vi "Periodic Tasks.vi"(8 "error in (no error)":errorcluster) -> ()   [LabVIEW 2014]
doc: "This VI runs in parallel to other tasks. It can contain as many user-defined periodic loops as you need. These can carry out PID or other sorts of timed response."
uses:
  <vilib>/Rock Robotics/WPI/DriverStation/WPI_DriverStationRobotMode2.ctl
  <vilib>/Utility/file.llb/Write To Spreadsheet File (string).vi
  <vilib>/Utility/file.llb/Write To Spreadsheet File (DBL).vi
  <vilib>/Rock Robotics/WPI/Joystick/WPI_JoystickGetSetRefNum.vi
  Robot Global Data.vi
  <vilib>/Rock Robotics/Network Tables/SD Read Boolean.vi
  <vilib>/Rock Robotics/Network Tables/SD Write Number.vi
  <vilib>/Rock Robotics/Network Tables/NT Write Number.vi
  <vilib>/Rock Robotics/Network Tables/SD Write Numeric Array.vi
  <vilib>/Rock Robotics/Network Tables/NT Read Boolean.vi
  <vilib>/Rock Robotics/Network Tables/NT Write Boolean.vi
  <vilib>/FPGAPlugInAG/roboRIO/niLvFpga_Close_roboRIO.vi
  <vilib>/Rock Robotics/SystemInterfaces/System/FPGA_SystemFPGA Ref Global.vi
  <vilib>/rvi/interface/nirviCloseFPGA/nirviCloseFPGA.xnode
  <vilib>/Rock Robotics/SystemInterfaces/System/FPGA_SystemFRC FPGA Ref.ctl
  <vilib>/Rock Robotics/SystemInterfaces/roboRIO_FPGA_2015_1.0.10.lvbitx
  navX-MXP-LabVIEW/navX-MXP Library/navX-MXP IMU.lvlib
  <vilib>/Rock Robotics/WPI/DriverStation/WPI_DriverStationAllianceInfo.ctl
  <vilib>/Rock Robotics/Network Tables/SD Read Number.vi
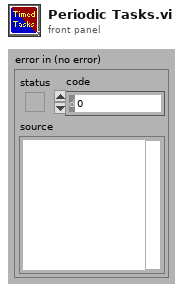
[diagram p1: front panel]
types:
  T1 = typedef "WPI_DriverStationRobotMode2.ctl" = enum16{"Autonomous Disabled", "Autonomous Enabled", "Teleop Disabled", "Teleop Enabled", "Disconnected", "Finish", "Test Disabled", "Test Enabled", "Emergency Stopped"}
  T2 = typedef "WPI_DriverStationPositionInfo.ctl" = enum16{"1", "2", "3"}
  T3 = typedef "WPI_DriverStationAllianceInfo.ctl" = enum16{"Red", "Blue", "Invalid"}
  T4 = typedef "WPI_MotorControlDeviceRef.ctl" = cluster{"DeviceStatus":errorcluster, "Type":T5, "PWM":cluster{"Controller":T6, "PWM Channel":T7, "DeadBand":T8}, "CAN":cluster{"Device Number":u8, "Control Mode":T9, "Semaphore":T10, "Max Vout":dbl, "TalonSRX Control Mode":T11}, "Invert":bool, "TransformRef":T12, "InvTransformRef":T12}
  T5 = typedef "WPI_MotorControlType.ctl" = enum16{"PWM", "CAN", "CANTalonSRX"}
  T6 = typedef "FPGA_TypedefDigitalModule.ctl" = enum16{"Controller 1"}
  T7 = typedef "FPGA_DIOPWMChannel.ctl" = enum8{"PWM 0", "PWM 1", "PWM 2", "PWM 3", "PWM 4", "PWM 5", "PWM 6", "PWM 7", "PWM 8", "PWM 9", "PWM MXP 0", "PWM MXP 1", "PWM MXP 2", "PWM MXP 3", "PWM MXP 4", "PWM MXP 5", "PWM MXP 6", "PWM MXP 7", "PWM MXP 8", "PWM MXP 9", "Invalid"}
  T8 = typedef "WPI_PWMDeadband.ctl" = cluster{"Name":string, "maxPositivePwm":i32, "minPositivePwm":i32, "centerPwm":i32, "maxNegativePwm":i32, "minNegativePwm":i32, "angularRange":u16}
  T9 = typedef "WPI_CANJaguar_ControlMode.ctl" = enum8{"Percent VBus", "Current", "Speed", "Position", "Voltage"}
  T10 = typedef "Semaphore RefNum" = refnum<k1>
  T11 = typedef "WPI_CANTalonSRX_APIControlMode.ctl" = enum8{"Percent VBus", "Speed", "Position", "Slave", "Unchanged / Invalid"}
  T12 = typedef "WPI_PWMTransform_ConPane.ctl" = refnum<vi>
  T13 = cluster{"FL Steering":T4, "FR Steering":T4, "RL Steering":T4, "RR Steering":T4}
  T14 = cluster{"FL Speed":T4, "FR Speed":T4, "RL Speed":T4, "RR Speed":T4}
  T15 = typedef "navX-MXP IMU.lvlib/navX Device TypeDef.ctl" = cluster{"navX Interface Protocol":T16, "navX Interface Protocol TypeDefs":cluster{"SPIDevRef":T17, "I2CDevRef":T19}, "navX System Information":cluster{"Board Information":T21, "Status":T22, "Offsets":T26}, "navX Common Information":cluster{"Update Rate (4Hz-60Hz)":T27, "refnum name":string, "error":errorcluster}}
  T16 = typedef "navX-MXP IMU.lvlib/navX Interface Protocol.ctl" = enum16{"SPI", "I2C"}
  T17 = typedef "WPI_SPIDevRef.ctl" = cluster{"DevStatus":errorcluster, "Handle":i32, "Controller":T6, "SPI Bus":T18}
  T18 = typedef "spi_bus.ctl" = enum16{"SPI On-Board, CS0", "SPI On-Board, CS1", "SPI On-Board, CS2", "SPI On-Board, CS3", "SPI MXP", "Invalid"}
  T19 = typedef "WPI_I2CDevRef.ctl" = cluster{"DevStatus":errorcluster, "Controller":T6, "Device Address":u8, "Handle":i32, "I2C Bus":T20}
  T20 = typedef "i2c_bus.ctl" = enum16{"I2C On-Board", "I2C MXP", "Invalid"}
  T21 = typedef "navX-MXP IMU.lvlib/navX Board Information.ctl" = cluster{"WhoAmI (50 | 0x32)":u8, "Board Revision":u8, "Firmware Major Version":u8, "Firmware Minor Version":u8}
  T22 = typedef "navX-MXP IMU.lvlib/navX Status Data.ctl" = cluster{"Update Rate Hz":u8, "Accelerometer Full-Scale Range":u8, "Gyro Full-Scale Range":u16, "NAVX_OP_STATUS":T23, "NAVX_CAL_STATUS":T24, "NAVX_SELFTEST_STATUS":u8, "NAVX_SENSOR_STATUS":T25}
  T23 = typedef "navX-MXP IMU.lvlib/navX NAVX_OP_STATUS.ctl" = u8
  T24 = typedef "navX-MXP IMU.lvlib/navX NAVX_CAL_STATUS.ctl" = u8
  T25 = typedef "navX-MXP IMU.lvlib/navX NAVX_SENSOR_STATUS.ctl" = cluster{"MOVING":bool, "YAW_STABLE":bool, "MAG_DISTURBANCE":bool, "ALTITUDE_VALID":bool, "SEALEVEL_PRESS_SET":bool, "FUSED_HEADING_VALID":bool}
  T26 = typedef "navX-MXP IMU.lvlib/navX Offsets Data.ctl" = cluster{"Yaw":dbl, "Quat W":dbl, "Quat X":dbl, "Quat Y":dbl, "Quat Z":dbl}
  T27 = typedef "navX-MXP IMU.lvlib/navX Update Rate.ctl" = u8
  T28 = typedef "navX-MXP IMU.lvlib/navX YPRH Data.ctl" = cluster{"Yaw":dbl, "Pitch":dbl, "Roll":dbl, "Heading":dbl}
  T29 = typedef "WPI_CANTalonSRX_GlobalStatus.ctl" = cluster{"Applied Throttle":dbl, "Module Enabled":bool, "CAN Error":errorcluster, "Closed Loop Error":dbl, "Forward Limit Switch Closed":bool, "Reverse Limit Switch Closed":bool, "Sensor Position":dbl, "Sensor Velocity":dbl, "Current":dbl, "Sticky Fault - Over Temp":bool, "Sticky Fault - Under Voltage":bool, "Sticky Fault - Forward Limit":bool, "Sticky Fault - Reverse Limit":bool, "Sticky Fault - Forward Soft Limit":bool, "Sticky Fault - Reverse Soft Limit":bool, "Brake is Enabled":bool, "Encoder Position":dbl, "Encoder Velocity":dbl, "Encoder Index Count":dbl, "Encoder A Pin State":bool, "Encoder B Pin State":bool, "Encoder Index Pin State":bool, "Analog In":dbl, "Analog In Velocity":dbl, "Temperature (C)":dbl, "Battery Voltage":dbl}
  T30 = cluster{"[0]":dbl, "[1]":dbl, "[2]":dbl, "[3]":dbl}
  T31 = typedef "FPGA_SystemFRC FPGA Ref.ctl" = refnum<k20>
  T32 = cluster{"refnum name":string, "refnum name":string, "refnum name":string, "refnum name":string}
  T33 = typedef "WPI_AnalogChannelDevRef.ctl" = cluster{"DevStatus":errorcluster, "Controller":T34, "Analog Channel":T35}
  T34 = typedef "FPGA_TypedefAnalogModule.ctl" = enum16{"Controller 1"}
  T35 = typedef "FPGA_AIChannel.ctl" = enum8{"AI 0", "AI 1", "AI 2", "AI 3", "AI MXP 0", "AI MXP 1", "AI MXP 2", "AI MXP 3", "Invalid"}
  T36 = typedef "WPI_JoystickDevRef.ctl" = cluster{"Device":T37}
  T37 = typedef "WPI_JoystickDeviceEnum.ctl" = enum16{"USB 0", "USB 1", "USB 2", "USB 3", "USB 4", "USB 5"}
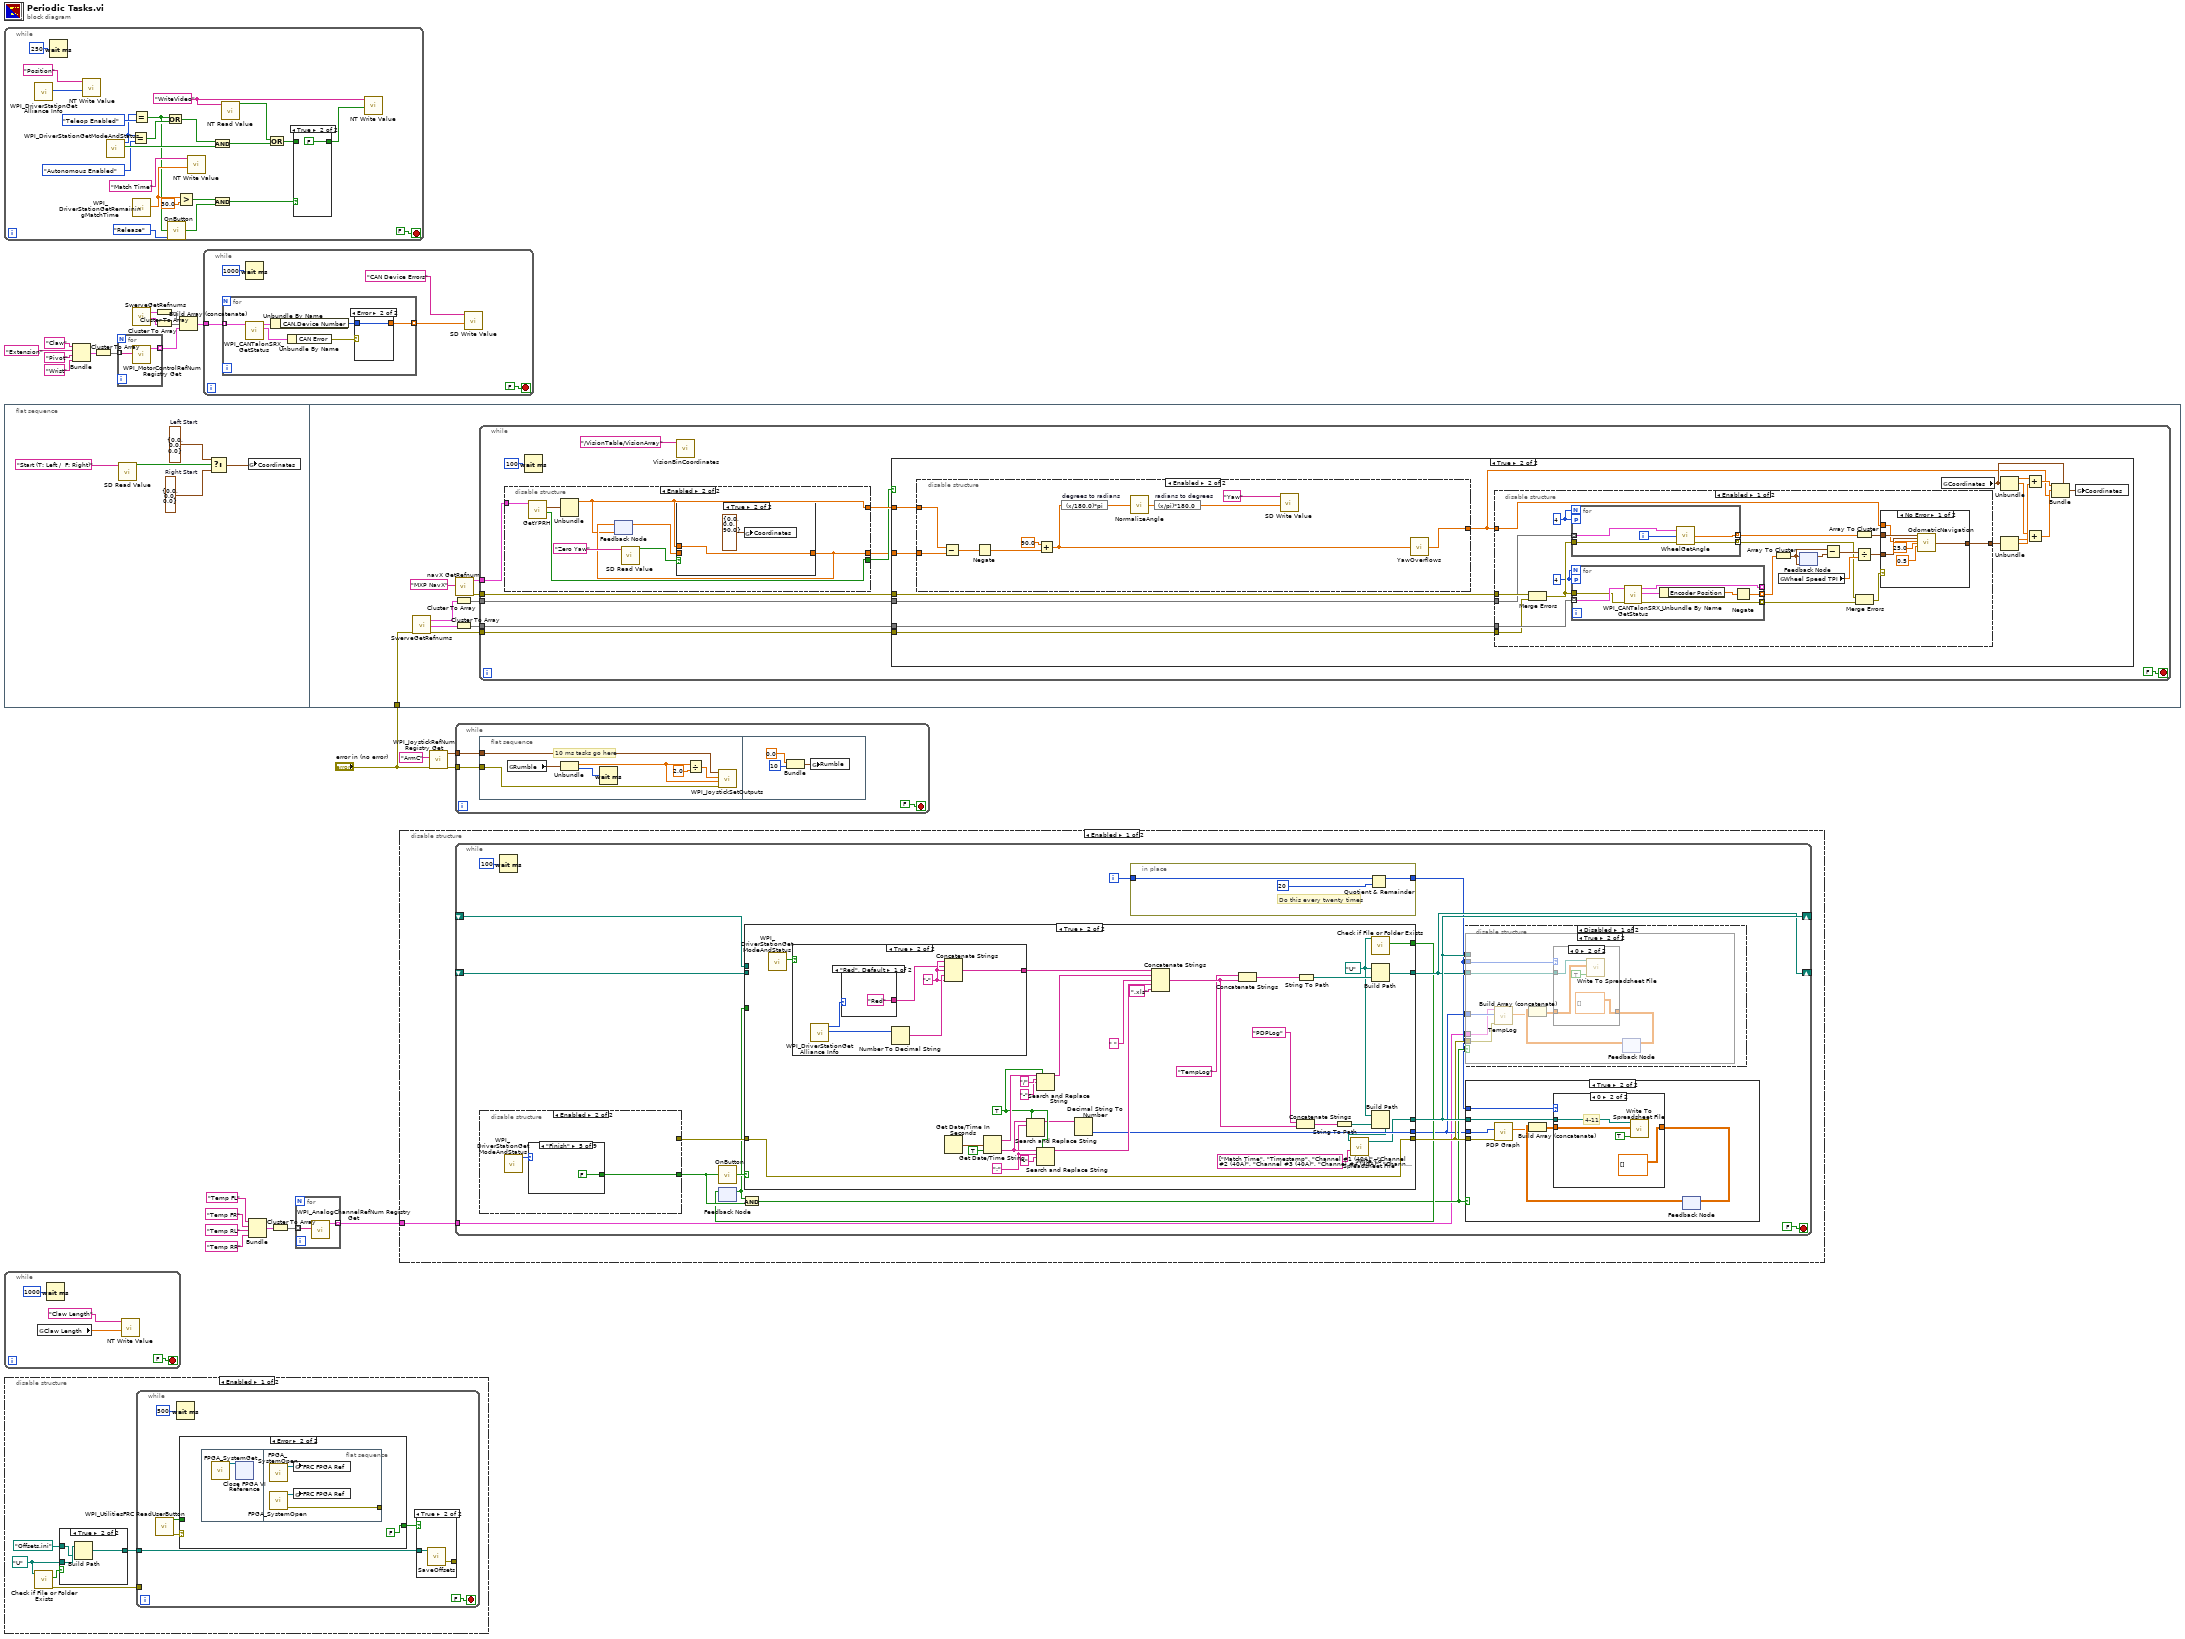
[diagram p0: block diagram]
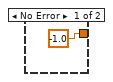
[diagram p3: hidden frame]
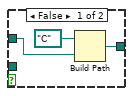
[diagram p4: hidden frame]
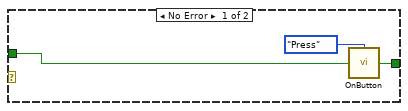
[diagram p5: hidden frame]
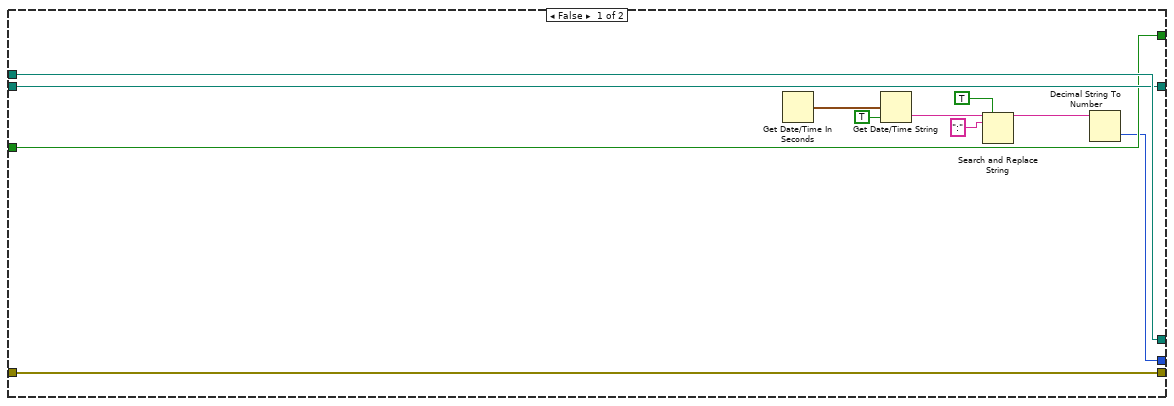
[diagram p11: hidden frame]
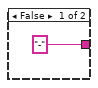
[diagram p12: hidden frame]
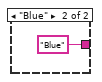
[diagram p13: hidden frame]
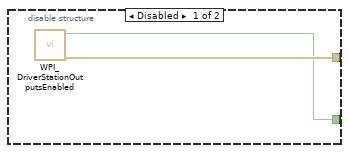
[diagram p16: hidden frame]
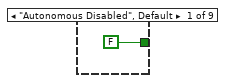
[diagram p17: hidden frame]
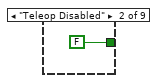
[diagram p18: hidden frame]
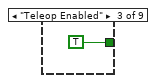
[diagram p19: hidden frame]
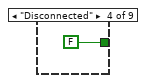
[diagram p20: hidden frame]
diagram:
  n1 = while {
    stop <- FALSE stop-if-true
    w43 = "WriteVideo" ("Name")
    n2 = call <vilib>:"WPI_DriverStationGet Alliance Info.vi"() -> ("Position"=w42:T2)  [unwired: 10 in, 1 out]
    n3 = Wait (ms)(milliseconds to wait=250) -> ()  [unwired: 1 out]
    n4 = call-poly <vilib>:"NT Write Value.vi"("Numeric"=w42, "Name"="Position") -> ()  [unwired: 9 in, 1 out]
    n5 = call <vilib>:"WPI_DriverStationGetModeAndStatus.vi"() -> ("FMS Attached"=w44:bool, "Robot Mode"=w28:T1)  [unwired: 10 in]
    n6 = Equal?(x=w28, y=WPI_DriverStationRobotMode2."Autonomous Enabled") -> (x = y?=w25:bool)
    n7 = Equal?(x=w28, y=WPI_DriverStationRobotMode2."Teleop Enabled" ("Robot Mode")) -> (x = y?=w24:bool)
    n8 = call <vilib>:"WPI_DriverStationGetRemainingMatchTime.vi"() -> ("Match Time(s)"=w31:sgl)  [unwired: 10 in, 1 out]
    n9 = Or(x=w24, y=w25) -> (x .or. y?=w26:bool)
    n10 = call "OnButton.vi"("Button"=w24, "Mode"=enum16{"Press", "Release", "Both"}."Release") -> ("Value"=w36:bool)
    n11 = Greater?(x=w31, y=sgl 30.0) -> (0:w33:bool)
    n12 = call-poly <vilib>:"NT Write Value.vi"("Numeric"=w31, "Name"="Match Time") -> ()  [unwired: 9 in, 1 out]
    n13 = And(x=w26, y=w44) -> (x .and. y?=w37:bool)
    n14 = And(x=w33, y=w36) -> (x .and. y?=w34:bool)
    n15 = call-poly <vilib>:"NT Read Value.vi"("Name"=w43) -> ("Boolean"=w38:bool)  [unwired: 9 in, 1 out]
    n16 = Or(x=w38, y=w37) -> (x .or. y?=w39:bool)
    n17 = case shown="True" w34 {
      tunnel: [w47 FALSE] -> w40
      tunnel: w39 -> [w47 _]
      frame False {
      }
      frame True {
      }
    }
    n18 = call-poly <vilib>:"NT Write Value.vi"("Boolean"=w40, "Name"=w43) -> ()  [unwired: 9 in, 1 out]
  }
  n19 = flat-sequence {
    tunnel: "error in (no error)" -> [w62]
    frame #0 {
      w49 = cluster{"X":dbl, "Y":dbl, "Heading":dbl} {"X"=0.0, "Y"=0.0, "Heading"=0.0}  # Left Start
      w50 = cluster{"X":dbl, "Y":dbl, "Heading":dbl} {"X"=0.0, "Y"=0.0, "Heading"=0.0}  # Right Start
      n20 = call-poly <vilib>:"SD Read Value.vi"("Name"="Start (T: Left /  F: Right)") -> ("Boolean"=w52:bool)  [unwired: 8 in, 2 out]
      n21 = Select(t=w49, s=w52, f=w50) -> (s? t:f=w51:cluster{"X":dbl, "Y":dbl, "Heading":dbl})
      n22 = global write "Robot Global Data.vi" "Coordinates"(w51) -> ()
    }
    frame #1 {
      n23 = call "SwerveGetRefnums.vi"("error in (no error)"=w62) -> ("Steering"=w55:T13, "Speed"=w57:T14, "error out"=w56:errorcluster)  [unwired: 8 in, 8 out]
      n24 = Cluster To Array(cluster=w55) -> (array=w54:T4[])
      n25 = Cluster To Array(cluster=w57) -> (array=w58:T4[])
      n26 = call "navX GetRefnum.vi"("refnum name"="MXP NavX") -> ("error out"=w59:errorcluster, "navX Device TypeDef"=w60:T15)  [unwired: 9 in]
      n27 = while {
        tunnel: w60 -> [w70]
        tunnel: w59 -> [w69]
        tunnel: w56 -> [w65]
        tunnel: w58 -> [w66]
        tunnel: w54 -> [w64]
        stop <- FALSE stop-if-true
        n28 = disable-structure shown="Enabled" {
          disable-tunnel: [w76 w77] -> w72
          disable-tunnel: [w75 w82] -> w71
          disable-tunnel: w70 -> [w74 w84]
          disable-tunnel: [_ w79] -> w68
          frame Disabled {
            n29 = call "GetFusedHeading.vi"("navX Device TypeDef"=w74) -> ("Valid?"=w75:bool, "Fused Heading"=w76:dbl)  [unwired: 8 in, 1 out]
          }
          frame Enabled {
            n30 = call "GetYPRH.vi"("navX Device TypeDef"=w84) -> ("Valid?"=w82:bool, "YPRH"=w83:T28)  [unwired: 8 in, 1 out]
            n31 = Unbundle(w83) -> ("Yaw"=w77:dbl)  [unwired: 3 out]
            n32 = feedback #1(w77) -> (w80:dbl)
            n33 = call-poly <vilib>:"SD Read Value.vi"("Name"="Zero Yaw") -> ("Boolean"=w78:bool)  [unwired: 8 in, 2 out]
            n34 = case shown="True" w78 {
              tunnel: w77 -> [_ w87]
              tunnel: [w85 w87] -> w79
              tunnel: w80 -> [w85 _]
              frame False {
              }
              frame True {
                n35 = global write "Robot Global Data.vi" "Coordinates"(cluster{"X":dbl, "Y":dbl, "Heading":dbl} {"X"=0.0, "Y"=0.0, "Heading"=90.0} ("Coordinates")) -> ()
              }
            }
            n36 = feedback-in #1(w79) -> ()
          }
        }
        n37 = Wait (ms)(milliseconds to wait=u32 100) -> ()  [unwired: 1 out]
        n38 = call "VisionBinCoordinates.vi"("Vision Array Name"="/VisionTable/VisionArray") -> ()  [unwired: 2 in, 3 out]
        n39 = case shown="True" w71 {
          tunnel: w72 -> [_ w95]
          tunnel: w69 -> [_ w94]
          tunnel: w68 -> [_ w93]
          tunnel: w66 -> [_ w91]
          tunnel: w65 -> [_ w90]
          tunnel: w64 -> [_ w89]
          frame False {
          }
          frame True {
            n40 = disable-structure shown="Enabled" {
              disable-tunnel: [w154 w156] -> w88
              disable-tunnel: w95 -> [w153 w165]
              disable-tunnel: w93 -> [_ w164]
              frame Disabled {
                # "Each time we enter, report that\nwe are running teleop"
                n41 = call-poly <vilib>:"SD Write Value.vi"("Numeric"=w153, "Name"="Fused Heading") -> ()  [unwired: 8 in, 2 out]
                n42 = call-poly <vilib>:"SD Read Value.vi"("Name"="Straight Forward Heading (on Red)") -> ("Numeric"=w146:dbl)  [unwired: 8 in, 2 out]
                n43 = call <vilib>:"WPI_DriverStationGet Alliance Info.vi"() -> ("Alliance"=w150:T3)  [unwired: 10 in, 1 out]
                n44 = Add(x=w146, y=90.0) -> (x+y=w144:dbl)
                n45 = Equal?(x=w150, y=WPI_DriverStationAllianceInfo."Blue") -> (x = y?=w148:bool)
                n46 = Subtract(x=w144, y=180.0) -> (x-y=w147:dbl)
                n47 = Select(t=w147, s=w148, f=w144) -> (s? t:f=w155:dbl)
                n48 = Subtract(x=w153, y=w155) -> (x-y=w154:dbl)
              }
              frame Enabled {
                n49 = Subtract(x=w165, y=w164) -> (x-y=w162:dbl)
                n50 = Negate(x=w162) -> (-x=w163:dbl)
                n51 = Add(x=90.0, y=w163) -> (x+y=w157:dbl)
                n52 = expression code="(x/180.0)*pi" "degrees to radians"(w157) -> (w158:dbl)
                n53 = call "NormalizeAngle.vi"("angle (rad)"=w158) -> ("angle (between pi and -pi)"=w160:dbl)
                n54 = expression code="(x/pi)*180.0" "radians to degrees"(w160) -> (w159:dbl)
                n55 = call-poly <vilib>:"SD Write Value.vi"("Numeric"=w159, "Name"="Yaw") -> ()  [unwired: 8 in, 2 out]
                n56 = call "YawOverflows.vi"("Yaw (degrees)"=w157) -> ("Yaw (with overflows)"=w156:dbl)
              }
            }
            n57 = disable-structure shown="Enabled" {
              disable-tunnel: w94 -> [w122 _]
              disable-tunnel: [w118 _] -> w92
              disable-tunnel: w91 -> [w123 _]
              disable-tunnel: w90 -> [w121 _]
              disable-tunnel: w89 -> [w109 _]
              disable-tunnel: w88 -> [w108 _]
              frame Enabled {
                w104 = 4
                w105 = 4
                n58 = Merge Errors(w122, w121) -> (w111:errorcluster)
                n59 = for {
                  N: w104 -> [_]
                  workers-P: w104 -> [_]
                  tunnel: w111 -> [w127]
                  tunnel: [w126] -> w110 mode=indexing
                  tunnel: w109 -> [w125] mode=indexing
                  tunnel: [w124] -> w106 mode=indexing
                  i -> [w128]
                  n60 = call "WheelGetAngle.vi"("error in (no error)"=w127, "Wheel"=w128, "CAN Talon SRX Ref"=w125) -> ("error out"=w126:errorcluster, "Sensor Position (rad)"=w124:dbl)  [unwired: 1 out]
                }
                n61 = for {
                  N: w105 -> [_]
                  tunnel: [w140] -> _ mode=indexing
                  tunnel: [w142] -> w120 mode=indexing
                  workers-P: w105 -> [_]
                  tunnel: w123 -> [w139] mode=indexing
                  tunnel: [w137] -> w113 mode=indexing
                  tunnel: w111 -> [w138]
                  n62 = call <vilib>:"WPI_CANTalonSRX_GetStatus.vi"("error in (no error)"=w138, "CAN Talon SRX Ref"=w139) -> ("error out"=w142:errorcluster, "Talon SRX Status"=w141:T29, "CAN Talon SRX Ref Out"=w140:T4)  [unwired: 7 in]
                  n63 = Unbundle By Name(w141) -> ("Encoder Position"=w136:dbl)
                  n64 = Negate(x=w136) -> (-x=w137:dbl)
                }
                n65 = Array To Cluster(array=w113) -> (cluster=w114:T30)
                n66 = global read "Robot Global Data.vi" "Wheel Speed TPI"() -> (w112:dbl)
                n67 = feedback #2(w114) -> (w115:T30)
                n68 = feedback-in #2(w114) -> ()
                n69 = Subtract(x=w114, y=w115) -> (x-y=w116:T30)
                n70 = Array To Cluster(array=w106) -> (cluster=w107:T30)
                n71 = Divide(x=w116, y=w112) -> (x/y=w117:T30)
                n72 = Merge Errors(w110, w120) -> (w119:errorcluster)
                n73 = case shown="No Error" w119 {
                  tunnel: [w132 cluster{"sy":dbl, "sx":dbl, "rot.":dbl} {"sy"=0.0, "sx"=0.0, "rot."=0.0} ("movement")] -> w118
                  tunnel: w117 -> [w134 _]
                  tunnel: w107 -> [w133 _]
                  tunnel: w108 -> [w129 _]
                  frame No Error {
                    n74 = call "OdometricNavigation.vi"("Wheel Angles (rad)"=w133, "Wheel Movements (in.)"=w134, "Robot angle (degrees)"=w129, "x and y error minimum (in.)"=25.0, "error minimum for rotation (rad)"=0.5 ("error minimum for rotation (in.)")) -> ("movement"=w132:cluster{"sy":dbl, "sx":dbl, "rot.":dbl})  [unwired: 14 in]
                  }
                  frame Error {
                  }
                }
              }
              frame Disabled {
              }
            }
            n75 = global read "Robot Global Data.vi" "Coordinates"() -> (w102:cluster{"X":dbl, "Y":dbl, "Heading":dbl})
            n76 = Unbundle(w102) -> ("X"=w101:dbl, "Y"=w98:dbl)  [unwired: 1 out]
            n77 = Unbundle(w92) -> ("sy"=w97:dbl, "sx"=w99:dbl)  [unwired: 1 out]
            n78 = Add(x=w101, y=w99) -> (x+y=w100:dbl)
            n79 = Add(x=w98, y=w97) -> (x+y=w96:dbl)
            n80 = Bundle(cluster=w102, "X"=w100, "Y"=w96, "Heading"=w88) -> (w103:cluster{"X":dbl, "Y":dbl, "Heading":dbl})
            n81 = global write "Robot Global Data.vi" "Coordinates"(w103) -> ()
          }
        }
      }
    }
  }
  n82 = while {
    stop <- FALSE stop-if-true
    n83 = global read "Robot Global Data.vi" "Claw Length"() -> (w167:dbl)
    n84 = Wait (ms)(milliseconds to wait=u32 1000) -> ()  [unwired: 1 out]
    n85 = call-poly <vilib>:"NT Write Value.vi"("Numeric"=w167, "Name"="Claw Length") -> ()  [unwired: 9 in, 1 out]
  }
  n86 = disable-structure shown="Enabled" {
    frame Enabled {
      w173 = path "U:/" ("base path")
      n87 = call <vilib>:"Check if File or Folder Exists.vi"("path"=w173) -> ("error out"=w171:errorcluster, "file or folder exists?"=w174:bool)  [unwired: 8 in, 1 out]
      n88 = case shown="True" w174 {
        tunnel: path "Offsets.ini" ("default name") -> [w178 w179]
        tunnel: [w177 w180] -> w172
        tunnel: w173 -> [_ w181]
        frame False {
          n89 = Build Path(base path=path "C:/", name or relative path=w178) -> (appended path=w177:path)
        }
        frame True {
          n90 = Build Path(base path=w181, name or relative path=w179) -> (appended path=w180:path)
        }
      }
      n91 = while {
        tunnel: w172 -> [w186]
        tunnel: w171 -> [_]
        stop <- FALSE stop-if-true
        n92 = call <vilib>:"WPI_UtilitiesFRC ReadUserButton.vi"() -> ("error out"=w184:errorcluster, "User Button"=w182:bool)  [unwired: 10 in]
        n93 = Wait (ms)(milliseconds to wait=u32 500) -> ()  [unwired: 1 out]
        n94 = case shown="Error" w184 {
          tunnel: w182 -> [w189 _]
          tunnel: [w190 FALSE ("Value")] -> w183
          frame No Error {
            n95 = call "OnButton.vi"("Button"=w189, "Mode"=enum16{"Press", "Release", "Both"}."Press") -> ("Value"=w190:bool)
          }
          frame Error {
            n96 = flat-sequence {
              tunnel: [w194] -> _
              frame #0 {
                n97 = call <vilib>:"FPGA_SystemGet.vi"() -> ("FRC FPGA Ref"=w192:T31)  [unwired: 11 in]
                n98 = xnode "Close FPGA VI Reference"("FPGA VI Reference In"=w192) -> ()  [unwired: 1 in, 1 out]
              }
              frame #1 {
                n99 = call <vilib>:"FPGA_SystemOpen.vi"() -> ("FRC FPGA Ref"=w193:T31)  [unwired: 1 in, 10 out]
                n100 = call <vilib>:"FPGA_SystemOpen.vi"() -> ("error out"=w194:errorcluster, "FRC FPGA Ref"=w195:T31)  [unwired: 1 in, 9 out]
                n101 = global write "FPGA_SystemFPGA Ref Global.vi" "FRC FPGA Ref"(w193) -> ()
                n102 = global write "FPGA_SystemFPGA Ref Global.vi" "FRC FPGA Ref"(w195) -> ()
              }
            }
          }
        }
        n103 = case shown="True" w183 {
          tunnel: w186 -> [_ w197]
          tunnel: [_ w196] -> _
          frame False {
          }
          frame True {
            n104 = call "SaveOffsets.vi"("configuration file path"=w197) -> ("error out"=w196:errorcluster)  [unwired: 3 in]
          }
        }
      }
    }
    frame Disabled {
    }
  }
  n105 = Bundle("Claw", "Extension", "Pivot", "Wrist") -> (w15:cluster{string, string, string, string})  [unwired: 1 in]
  n106 = Cluster To Array(cluster=w15) -> (array=w10:string[])
  n107 = for {
    tunnel: w10 -> [w199] mode=indexing
    tunnel: [w198] -> w9 mode=indexing
    n108 = call <vilib>:"WPI_MotorControlRefNum Registry Get.vi"("refnum name"=w199) -> ("MotorControlDevRef"=w198:T4)  [unwired: 9 in, 1 out]
  }
  n109 = call "SwerveGetRefnums.vi"() -> ("Steering"=w8:T13, "Speed"=w7:T14)  [unwired: 9 in, 9 out]
  n110 = Cluster To Array(cluster=w8) -> (array=w5:T4[])
  n111 = Cluster To Array(cluster=w7) -> (array=w6:T4[])
  n112 = Build Array (concatenate)(w5, w6, w9) -> (w4:T4[])
  n113 = while {
    tunnel: w4 -> [w203]
    stop <- FALSE stop-if-true
    n114 = for {
      tunnel: w203 -> [w209] mode=indexing
      tunnel: [w205] -> w201 mode=indexing
      n115 = call <vilib>:"WPI_CANTalonSRX_GetStatus.vi"("CAN Talon SRX Ref"=w209) -> ("Talon SRX Status"=w210:T29, "CAN Talon SRX Ref Out"=w208:T4)  [unwired: 8 in, 1 out]
      n116 = Unbundle By Name(w208) -> ("CAN.Device Number"=w207:u8)
      n117 = Unbundle By Name(w210) -> ("CAN Error"=w206:errorcluster)
      n118 = case shown="Error" w206 {
        tunnel: w207 -> [_ w212]
        tunnel: [-1.0 w212] -> w205
        frame No Error {
        }
        frame Error {
        }
      }
    }
    n119 = Wait (ms)(milliseconds to wait=u32 1000) -> ()  [unwired: 1 out]
    n120 = call-poly <vilib>:"SD Write Value.vi"("Numeric Array"=w201, "Name"="CAN Device Errors") -> ()  [unwired: 8 in, 2 out]
  }
  n121 = Bundle("refnum name"="Temp FL", "refnum name"="Temp FR", "refnum name"="Temp RL", "refnum name"="Temp RR") -> (w21:T32)  [unwired: 1 in]
  n122 = Cluster To Array(cluster=w21) -> (array=w22:string[])
  n123 = for {
    tunnel: w22 -> [w214] mode=indexing
    tunnel: [w213] -> w16 mode=indexing
    n124 = call <vilib>:"WPI_AnalogChannelRefNum Registry Get.vi"("refnum name"=w214) -> ("AIDeviceRef"=w213:T33)  [unwired: 9 in, 1 out]
  }
  n125 = disable-structure shown="Enabled" {
    disable-tunnel: w16 -> [w215 _]
    frame Enabled {
      n126 = while {
        shift-right: [w231] -> _
        shift-left: _ -> [w230]
        shift-right: [w227] -> _
        shift-left: _ -> [w226]
        tunnel: w215 -> [w216]
        i -> [w219]
        stop <- FALSE stop-if-true
        n127 = disable-structure shown="Enabled" {
          disable-tunnel: [w321 w323] -> w224
          disable-tunnel: [w322 _] -> w228
          frame Disabled {
            n128 = call <vilib>:"WPI_DriverStationOutputsEnabled.vi"() -> ("error out"=w322:errorcluster, "OutputsEnabled?"=w321:bool)  [unwired: 10 in]
          }
          frame Enabled {
            n129 = call <vilib>:"WPI_DriverStationGetModeAndStatus.vi"() -> ("Robot Mode"=w324:T1)  [unwired: 10 in, 1 out]
            n130 = case shown="\"Finish\"" w324 {
              tunnel: [FALSE FALSE TRUE FALSE FALSE FALSE TRUE FALSE TRUE] -> w323
              frame "Autonomous Disabled", Default {
              }
              frame "Teleop Disabled" {
              }
              frame "Teleop Enabled" {
              }
              frame "Disconnected" {
              }
              frame "Finish" {
              }
              frame "Test Disabled" {
              }
              frame "Test Enabled" {
              }
              frame "Emergency Stopped" {
              }
              frame "Autonomous Enabled" {
              }
            }
          }
        }
        n131 = Wait (ms)(milliseconds to wait=u32 100) -> ()  [unwired: 1 out]
        n132 = call "OnButton.vi"("Button"=w224) -> ("Value"=w232:bool)  [unwired: 1 in]
        n133 = feedback #3() -> (w220:bool)  [unwired: 1 in]
        n134 = And(x=w220, y=w224) -> (x .and. y?=w221:bool)
        n135 = case shown="True" w232 {
          tunnel: [w264 w266] -> w231
          tunnel: w230 -> [w264 _]
          tunnel: [w263 w272] -> w225
          tunnel: w228 -> [w263 w272]
          tunnel: [w262 w283] -> w227
          tunnel: w226 -> [w262 _]
          tunnel: [w261 w271] -> w222
          tunnel: w220 -> [w261 _]
          tunnel: [w260 w270] -> w217
          frame False {
            n136 = Get Date/Time In Seconds() -> (seconds since 1Jan1904=w256:timestamp)
            n137 = Get Date/Time String(seconds (now)=w256, want seconds? (F)=TRUE) -> (time string=w258:string)  [unwired: 1 in, 1 out]
            n138 = Search and Replace String(replace all?=TRUE ("replace all? (F)"), input string=w258, search string=":") -> (result string=w259:string)  [unwired: 5 in, 3 out]
            n139 = Decimal String To Number(string=w259) -> (number=w260:i32)  [unwired: 2 in, 1 out]
          }
          frame True {
            w277 = ":" ("search string")
            w276 = TRUE ("replace all? (F)")
            w285 = path "U:/" ("base path")
            n140 = call <vilib>:"WPI_DriverStationGetModeAndStatus.vi"() -> ("FMS Attached"=w295:bool)  [unwired: 10 in, 1 out]
            n141 = case shown="True" w295 {
              tunnel: ["-" ("string") w299] -> w294
              frame False {
              }
              frame True {
                w300 = "-" ("string")
                n142 = call <vilib>:"WPI_DriverStationGet Alliance Info.vi"() -> ("Position"=w302:T2, "Alliance"=w297:T3)  [unwired: 10 in]
                n143 = case shown="\"Red\", Default" w297 {
                  tunnel: ["Red" "Blue"] -> w298
                  frame "Red", Default {
                  }
                  frame "Blue" {
                  }
                }
                n144 = Number To Decimal String(number=w302) -> (decimal integer string=w301:string)  [unwired: 1 in]
                n145 = Concatenate Strings(w300, w298, w300, w301, w300) -> (w299:string)
              }
            }
            n146 = Get Date/Time In Seconds() -> (seconds since 1Jan1904=w292:timestamp)
            n147 = Get Date/Time String(seconds (now)=w292, want seconds? (F)=TRUE) -> (date string=w282:string, time string=w278:string)  [unwired: 1 in]
            n148 = Search and Replace String(replace all?=w276, input string=w278, search string=w277) -> (result string=w269:string)  [unwired: 5 in, 3 out]
            n149 = Search and Replace String(replace all?=w276, input string=w282, search string="/", replace string="-" ("replace string (\"\")")) -> (result string=w279:string)  [unwired: 4 in, 3 out]
            n150 = Search and Replace String(replace all?=w276, input string=w278, search string=w277, replace string="-") -> (result string=w275:string)  [unwired: 4 in, 3 out]
            n151 = Decimal String To Number(string=w269) -> (number=w270:i32)  [unwired: 2 in, 1 out]
            n152 = Concatenate Strings(w294, w279, " " ("string"), w275, ".xls" ("string")) -> (w288:string)
            n153 = Concatenate Strings("TempLog" ("string"), w288) -> (w287:string)
            n154 = Concatenate Strings("PDPLog", w288) -> (w290:string)
            n155 = String To Path(string=w287) -> (path=w286:path)
            n156 = String To Path(string=w290) -> (path=w293:path)
            n157 = call <vilib>:"Check if File or Folder Exists.vi"("path"=w285) -> ("file or folder exists?"=w271:bool)  [unwired: 8 in, 2 out]
            n158 = Build Path(base path=w285, name or relative path=w286) -> (appended path=w283:path)
            n159 = Build Path(base path=w285, name or relative path=w293) -> (appended path=w267:path)
            n160 = call-poly <vilib>:"Write To Spreadsheet File.vi"("1D data"=string[] ["Match Time", "Timestamp", "Channel #1 (40A)", "Channel #2 (40A)", "Channel #3 (40A)", "Channel #4 (40A)", "Channel #13 (40A)", "Channel #14 (40A)", "Channel #15 (40A)", "Channel #16 (40A)", "Channel #5 (20/30A)", "Channel #6 (20/30A)", "Channel #7 (20/30A)", "Channel #8 (20/30A)", "Channel #9 (20/30A)", "Channel #10 (20/30A)", "Channel #11 (20/30A)", "Channel #12 (20/30A)", "PDP Voltage"] ("appended array"), "file path (dialog if empty)"=w267) -> ("new file path (Not A Path if cancelled)"=w266:path)  [unwired: 6 in]
          }
        }
        n161 = feedback-in #3(w222) -> ()
        n162 = in-place {
          in-place-border: w219 -> [w307]
          in-place-border: [w306] -> w218
          # "Do this every twenty times"
          n163 = Quotient & Remainder(x=w307, y=20) -> (x-y*floor(x/y)=w306:i32)  [unwired: 1 out]
        }
        n164 = disable-structure shown="Disabled" {
          disable-tunnel: w231 -> [w239 _]
          disable-tunnel: w227 -> [w238 _]
          disable-tunnel: w225 -> [w237 _]
          disable-tunnel: w221 -> [w236 _]
          disable-tunnel: w218 -> [w235 _]
          disable-tunnel: w217 -> [w234 _]
          disable-tunnel: w216 -> [w233 _]
          frame Disabled {
            n165 = case shown="True" w236 {
              tunnel: w237 -> [_ w245]
              tunnel: w238 -> [_ w243]
              tunnel: w239 -> [_ _]
              tunnel: w235 -> [_ w248]
              tunnel: w234 -> [_ w247]
              tunnel: w233 -> [_ w244]
              frame False {
              }
              frame True {
                n166 = call "TempLog.vi"("error in (no error)"=w245, "Timestamp"=w247, "Temp Refs"=w244) -> ("Temp"=w240:dbl[])  [unwired: 7 in, 1 out]
                n167 = feedback #4() -> (w241:dbl[][])  [unwired: 1 in]
                n168 = Build Array (concatenate)(w241, w240) -> (w242:dbl[][])
                n169 = case shown="0" w248 {
                  tunnel: w243 -> [_ w253]
                  tunnel: w242 -> [w249 w251]
                  tunnel: [w249 dbl[][] []] -> w246
                  frame 1, Default {
                  }
                  frame 0 {
                    n170 = call-poly <vilib>:"Write To Spreadsheet File.vi"("append to file? (new file:F)"=TRUE, "2D data"=w251, "file path (dialog if empty)"=w253) -> ()  [unwired: 5 in, 1 out]
                  }
                }
                n171 = feedback-in #4(w246) -> ()
              }
            }
          }
          frame Enabled {
          }
        }
        n172 = case shown="True" w221 {
          tunnel: w225 -> [_ w315]
          tunnel: w231 -> [_ w314]
          tunnel: w217 -> [_ w312]
          tunnel: w218 -> [_ w311]
          frame False {
          }
          frame True {
            n173 = call "PDP Graph.vi"("error in"=w315, "Timestamp"=w312) -> ("Current"=w308:dbl[])  [unwired: 8 in, 1 out]
            n174 = feedback #5() -> (w309:dbl[][])  [unwired: 1 in]
            n175 = Build Array (concatenate)(w309, w308) -> (w310:dbl[][])
            n176 = case shown="0" w311 {
              tunnel: w314 -> [_ w320]
              tunnel: w310 -> [w316 w318]
              tunnel: [w316 dbl[][] []] -> w313
              frame 1, Default {
              }
              frame 0 {
                # "4-11"
                n177 = call-poly <vilib>:"Write To Spreadsheet File.vi"("append to file? (new file:F)"=TRUE, "2D data"=w318, "file path (dialog if empty)"=w320) -> ()  [unwired: 5 in, 1 out]
              }
            }
            n178 = feedback-in #5(w313) -> ()
          }
        }
      }
    }
    frame Disabled {
    }
  }
  n179 = call <vilib>:"WPI_JoystickRefNum Registry Get.vi"("error in (no error)"="error in (no error)", "refnum name"="ArmC") -> ("error out"=w3:errorcluster, "JoystickDevRef"=w1:T36)  [unwired: 8 in]
  n180 = while {
    tunnel: w3 -> [w335]
    tunnel: w1 -> [w334]
    stop <- FALSE stop-if-true
    n181 = flat-sequence {
      tunnel: w335 -> [w341]
      tunnel: w334 -> [w340]
      frame #0 {
        # "10 ms tasks go here"
        n182 = global read "Robot Global Data.vi" "Rumble"() -> (w339:cluster{"Intensity":dbl, "Duration":i16})
        n183 = Unbundle(w339) -> ("Intensity"=w338:dbl, "Duration"=w337:i16)
        n184 = Wait (ms)(milliseconds to wait=w337) -> ()  [unwired: 1 out]
        n185 = Divide(x=w338, y=2.0) -> (x/y=w342:dbl)
        n186 = call <vilib>:"WPI_JoystickSetOutputs.vi"("error in (no error)"=w341, "Right Rumble"=w338, "Left Rumble"=w342, "JoystickDevRef"=w340) -> ()  [unwired: 6 in, 2 out]
      }
      frame #1 {
        n187 = Bundle("t"=0.0, "f"=i16 10) -> (w344:cluster{"t":dbl, "f":i16})  [unwired: 1 in]
        n188 = global write "Robot Global Data.vi" "Rumble"(w344) -> ()
      }
    }
  }
